vi "Write.vi"(6 "Type":T1=enum."SGL" format="%.0x", 7 "Register":u16=25472 format="%x", 8 "error in":errorcluster, 10 "Data":variant, 11 "Red-y Pressure Control CFG in":refnum<class "Red-y Pressure Control CFG.lvclass">) -> (0 "error out":errorcluster, 3 "Red-y Pressure Control CFG out":refnum<class "Red-y Pressure Control CFG.lvclass">)   [LabVIEW 2023, in "Red-y Pressure Control CFG.lvclass"]
uses:
  Red-y Pressure Control CFG.lvclass
  Red-y Pressure Control CFG.lvclass/Red-y Pressure Control CFG.ctl
  <userlib>/_OpenG.lib/lvdata/lvdata.llb/Type Descriptor Enumeration__ogtk.ctl
  <userlib>/_OpenG.lib/lvdata/lvdata.llb/openg_variant.lvlib
  Read Write PE Input.ctl
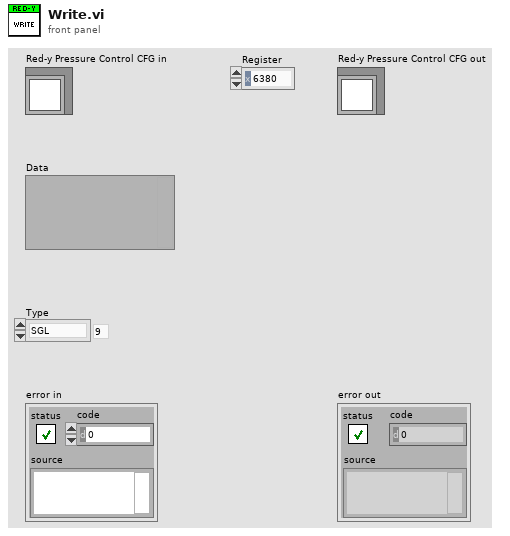
[diagram p1: front panel]
types:
  T1 = typedef "openg_variant.lvlib/Type Descriptor Enumeration__ogtk.ctl" = enum8{"<Null>", "I8", "I16", "I32", "I64", "U8", "U16", "U32", "U64", "SGL", "DBL", "EXT", "CSG", "CDB", "CXT", "0x0F", "0x10", "0x11", "0x12", "0x13", "0x14", "Enum U8", "Enum U16", "Enum U32", "Enum U64", "SGL PQ", "DBL PQ", "EXT PQ", "CSG PQ", "CDB PQ", "CXT PQ", "0x1F", "0x20", "Boolean", "0x22", "0x23", "0x24", "0x25", "0x26", "0x27", "0x28", "0x29", "0x2A", "0x2B", "0x2C", "0x2D", "0x2E", "0x2F", "String", "0x31", "Path", "Pict", "0x34", "0x35", "0x36", "DAQ", "0x38", "0x39", "0x3A", "0x3B", "0x3C", "0x3D", "0x3E", "0x3F", "Array", "0x41", "0x42", "0x43", "0x44", "0x45", "0x46", "0x47", "0x48", "0x49", "0x4A", "0x4B", "0x4C", "0x4D", "0x4E", "0x4F", "Cluster", "0x51", "0x52", "Variant", "Waveform", "0x55", "0x56", "0x57", "0x58", "0x59", "0x5A", "0x5B", "0x5C", "0x5D", "0x5E", "Fixed Point", "0x60", "0x61", "0x62", "0x63", "0x64", "0x65", "0x66", "0x67", "0x68", "0x69", "0x6A", "0x6B", "0x6C", "0x6D", "0x6E", "0x6F", "Refnum", "0x71", "0x72", "Set Collection", "Map Collection"}
  T2 = typedef "Read Write PE Input.ctl" = cluster{"Action":enum16{"Write", "Read"}, "Register":u16, "Type":T1, "Data":variant}
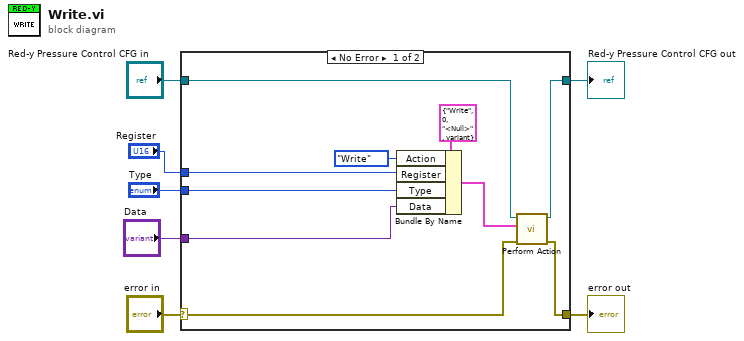
[diagram p0: block diagram]
diagram:
  n1 = case shown="No Error" "error in" {
    selector: "error in" -> [w14 w19]
    tunnel: [w13 w19] -> w6
    tunnel: [w11 w18] -> w4
    tunnel: "Red-y Pressure Control CFG in" -> [w12 w18]
    tunnel: "Register" -> [w10 _]
    tunnel: "Type" -> [w9 _]
    tunnel: "Data" -> [w8 _]
    frame No Error {
      n2 = Bundle By Name(cluster=T2 {"Action"=enum."Write", "Register"=0, "Type"=enum."<Null>", "Data"=variant}, "Action"=enum16{"Write", "Read"}."Write", "Register"=w10, "Type"=w9, "Data"=w8) -> (w16:T2)
      n3 = call-dynamic "Perform Action.vi"("error in"=w14, "Input"=w16, "Red-y Read Write CFG in"=w12) -> ("error out"=w13:errorcluster, "Red-y Read Write CFG out"=w11:refnum<class "Red-y Pressure Control CFG.lvclass">)  [unwired: 6 in, 1 out]
    }
    frame Error {
    }
  }
  "error out" <- w6
  "Red-y Pressure Control CFG out" <- w4
